vi "ReplaceScanFunc.vi"(0 "LoadedInstIn":refnum<class "BaseDevice.lvclass">[](array[class]), 1 "LoadedFuncArr":string[](array[string]), 2 "ScanFunc":string, 5 "ScanSubPan":refnum<vi>, 7 "WholeTask(No:T)":bool, 9 "ScanFuncArrIn":string[][](array[string]), 11 "ErrorIn(No Error)":errorcluster caption="entrée d'erreur (pas d'erreur)", 12 "ActScanPar":bool[](array[boolean]), 13 "TaskIdx":i32) -> (4 "LoadedInst":refnum<class "BaseDevice.lvclass">[](array[class]), 10 "ScanFuncArrOut":string[][](array[string]), 14 "ActScanParOut":bool[](array[boolean]), 15 "sortie d'erreur":errorcluster)   [LabVIEW 2019]
uses:
  DevicesClass/BaseDevice/BaseDevice.lvclass
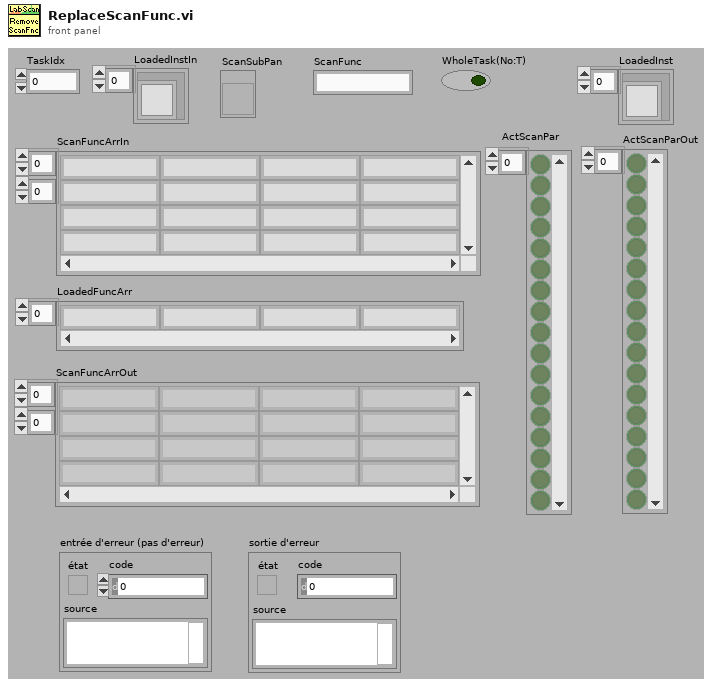
[diagram p1: front panel]
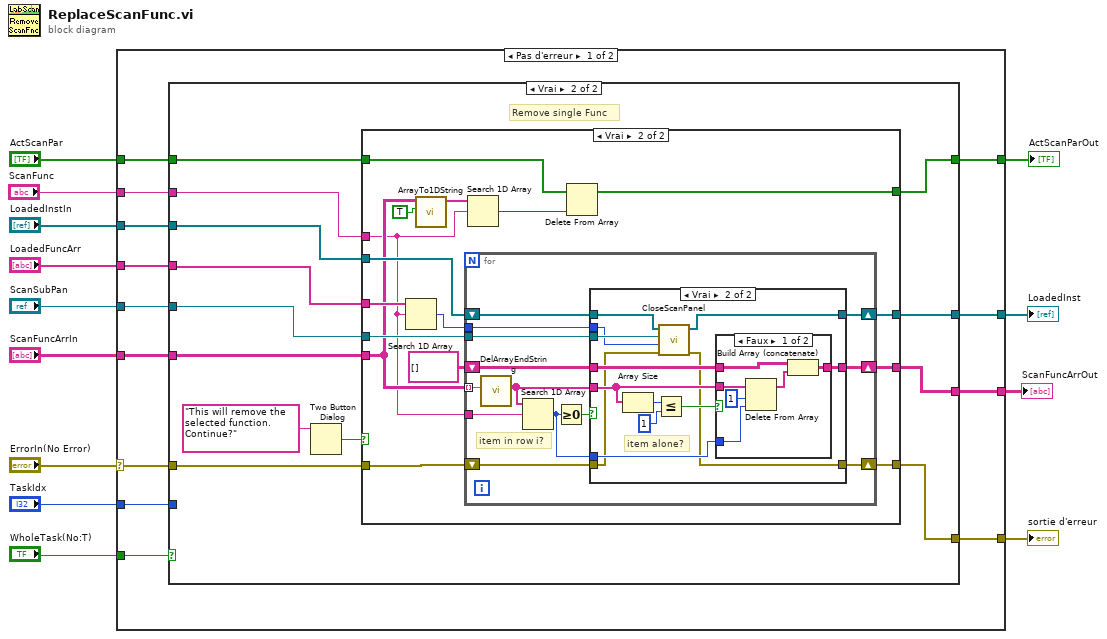
[diagram p0: block diagram]
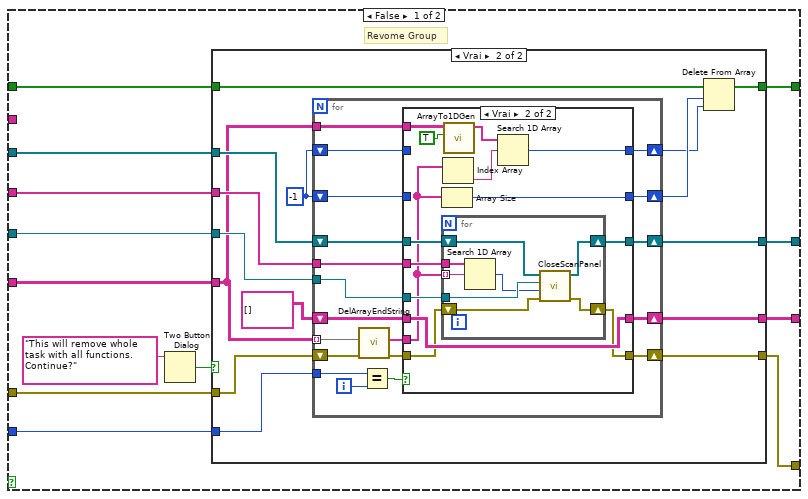
[diagram p2: hidden frame]
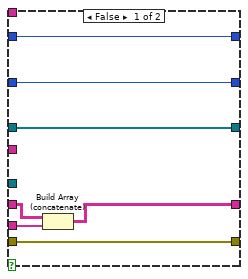
[diagram p4: hidden frame]
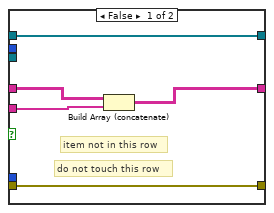
[diagram p6: hidden frame]
diagram:
  n1 = case shown="Pas d'erreur" "ErrorIn(No Error)" {
    selector: "ErrorIn(No Error)" -> [w26 w181]
    tunnel: "ScanFuncArrIn" -> [w23 w180]
    tunnel: "WholeTask(No:T)" -> [w24 _]
    tunnel: [w20 w181] -> w10
    tunnel: [w21 w180] -> w9
    tunnel: "ActScanPar" -> [w17 w179]
    tunnel: [w14 w179] -> w7
    tunnel: "TaskIdx" -> [w25 _]
    tunnel: [w22 w178] -> w5
    tunnel: "LoadedInstIn" -> [w19 w178]
    tunnel: "LoadedFuncArr" -> [w18 _]
    tunnel: "ScanSubPan" -> [w16 _]
    tunnel: "ScanFunc" -> [w15 _]
    frame No Error {
      n2 = case shown="Vrai" w24 {
        tunnel: w23 -> [w36 w116]
        tunnel: w25 -> [w35 _]
        tunnel: w17 -> [w28 w110]
        tunnel: w26 -> [w38 w112]
        tunnel: [w34 w119] -> w22
        tunnel: [w33 w118] -> w21
        tunnel: [w32 w117] -> w20
        tunnel: w19 -> [w30 w114]
        tunnel: w18 -> [w31 w113]
        tunnel: w16 -> [w29 w115]
        tunnel: w15 -> [_ w111]
        tunnel: [w27 w109] -> w14
        frame False {
          # "Revome Group"
          n3 = Two Button Dialog(message="This will remove whole task with all functions. Continue?") -> (T button?=w37:bool)  [unwired: 2 in]
          n4 = case shown="Vrai" w37 {
            tunnel: w36 -> [w43 w46]
            tunnel: w35 -> [_ w51]
            tunnel: [w43 w57] -> w33
            tunnel: w38 -> [w42 w58]
            tunnel: [w42 w56] -> w32
            tunnel: w30 -> [w41 w52]
            tunnel: w29 -> [_ w55]
            tunnel: w31 -> [_ w54]
            tunnel: [w41 w53] -> w34
            tunnel: w28 -> [w40 w50]
            tunnel: [w40 w48] -> w27
            frame False {
              # "canceled"
            }
            frame True {
              w45 = -1
              n5 = for {
                tunnel: w46 -> [w74] mode=indexing
                shift-right: [w70] -> w57
                shift-left: string[][] [] -> [w71]
                tunnel: w51 -> [w75]
                shift-right: [w69] -> w56
                shift-left: w58 -> [w77]
                tunnel: w55 -> [w67]
                tunnel: w54 -> [w66]
                shift-right: [w65] -> w53
                shift-left: w52 -> [w64]
                shift-right: [w63] -> w49
                shift-left: w45 -> [w62]
                tunnel: w46 -> [w61]
                shift-right: [w60] -> w44
                shift-left: w45 -> [w59]
                i -> [w76]
                n6 = call <userlib>:"DelArrayEndString.vi"("ErrorIn(No Error)"=w77, "Array In"=w74) -> ("sortie d'erreur"=w68:errorcluster, "Array Out"=w72:string[])  [unwired: 8 in]
                n7 = Equal?(x=w75, y=w76) -> (x = y?=w73:bool)
                n8 = case shown="Vrai" w73 {
                  tunnel: w72 -> [w84 w90]
                  tunnel: w71 -> [w83 w97]
                  tunnel: [w82 w97] -> w70
                  tunnel: [w81 w93] -> w69
                  tunnel: w68 -> [w81 w94]
                  tunnel: w64 -> [w80 w95]
                  tunnel: w67 -> [_ w96]
                  tunnel: w66 -> [_ w98]
                  tunnel: [w80 w92] -> w65
                  tunnel: [w79 w91] -> w63
                  tunnel: w62 -> [w79 _]
                  tunnel: w61 -> [_ w89]
                  tunnel: [w78 w85] -> w60
                  tunnel: w59 -> [w78 _]
                  frame False {
                    n9 = Build Array (concatenate)(w83, w84) -> (w82:string[][])
                  }
                  frame True {
                    n10 = Array Size(array=w90) -> (size(s)=w91:i32)
                    n11 = for {
                      tunnel: w98 -> [w99]
                      tunnel: w90 -> [w106] mode=indexing
                      tunnel: w96 -> [w103]
                      shift-right: [w104] -> w93
                      shift-left: w94 -> [w105]
                      shift-right: [w100] -> w92
                      shift-left: w95 -> [w101]
                      n12 = Search 1D Array(1D array=w99, element=w106) -> (index of element=w102:i32)  [unwired: 1 in]
                      n13 = call "CloseScanPanel.vi"("error in (no error)"=w105, "Index"=w102, "SubPanRef"=w103, "LoadedInst"=w101) -> ("sortie d'erreur"=w104:errorcluster, "LoadedInst Out"=w100:refnum<class "BaseDevice.lvclass">[])  [unwired: 6 in]
                    }
                    n14 = Index Array(array=w90) -> (element=w86:string)  [unwired: 1 in]
                    n15 = call-poly <userlib>:"ArrayTo1DGen.vi"("DelArrEnd(F)"=TRUE, "tableau"=w89) -> ("Array Out"=w87:string[])  [unwired: 7 in, 2 out]
                    n16 = Search 1D Array(1D array=w87, element=w86) -> (index of element=w85:i32)  [unwired: 1 in]
                  }
                }
              }
              n17 = Delete From Array(array=w50, length=w49, index=w44) -> (array with subset deleted=w48:bool[])  [unwired: 1 out]
            }
          }
        }
        frame True {
          # "Remove single Func"
          n18 = Two Button Dialog(message="This will remove the selected function. Continue?") -> (T button?=w107:bool)  [unwired: 2 in]
          n19 = case shown="Vrai" w107 {
            tunnel: w116 -> [w120 w131]
            tunnel: [w120 w138] -> w118
            tunnel: w111 -> [_ w129]
            tunnel: w114 -> [w123 w137]
            tunnel: w115 -> [_ w136]
            tunnel: w113 -> [_ w135]
            tunnel: [w121 w133] -> w117
            tunnel: [w123 w132] -> w119
            tunnel: w112 -> [w121 w128]
            tunnel: w110 -> [w122 w127]
            tunnel: [w122 w126] -> w109
            frame False {
              # "canceled"
            }
            frame True {
              n20 = Search 1D Array(1D array=w135, element=w129) -> (index of element=w134:i32)  [unwired: 1 in]
              n21 = call <userlib>:"ArrayTo1DString.vi"("DelArrEnd(F)"=TRUE, "tableau"=w131) -> ("Array Out"=w130:string[])  [unwired: 7 in, 2 out]
              n22 = for {
                tunnel: w131 -> [w150] mode=indexing
                tunnel: w129 -> [w152]
                shift-right: [w147] -> w138
                shift-left: string[][] [] -> [w148]
                tunnel: w136 -> [w145]
                tunnel: w134 -> [w143]
                shift-right: [w141] -> w133
                shift-left: w128 -> [w142]
                shift-right: [w140] -> w132
                shift-left: w137 -> [w146]
                # "item in row i?"
                n23 = call <userlib>:"DelArrayEndString.vi"("Array In"=w150) -> ("Array Out"=w149:string[])  [unwired: 9 in, 1 out]
                n24 = Search 1D Array(1D array=w149, element=w152) -> (index of element=w144:i32)  [unwired: 1 in]
                n25 = Greater Or Equal To 0?(x=w144) -> (x >= 0?=w151:bool)
                n26 = case shown="Vrai" w151 {
                  tunnel: [w156 w166] -> w147
                  tunnel: w149 -> [w157 w165]
                  tunnel: w148 -> [w155 w167]
                  tunnel: w146 -> [w153 w160]
                  tunnel: w145 -> [_ w163]
                  tunnel: w144 -> [_ w164]
                  tunnel: w143 -> [_ w159]
                  tunnel: w142 -> [w154 w162]
                  tunnel: [w154 w161] -> w141
                  tunnel: [w153 w158] -> w140
                  frame False {
                    # "item not in this row"
                    # "do not touch this row"
                    n27 = Build Array (concatenate)(w155, w157) -> (w156:string[][])
                  }
                  frame True {
                    # "item alone?"
                    n28 = Array Size(array=w165) -> (size(s)=w170:i32)
                    n29 = Less Or Equal?(x=w170, y=1) -> (x <= y?=w168:bool)
                    n30 = call "CloseScanPanel.vi"("error in (no error)"=w162, "Index"=w159, "SubPanRef"=w163, "LoadedInst"=w160) -> ("sortie d'erreur"=w161:errorcluster, "LoadedInst Out"=w158:refnum<class "BaseDevice.lvclass">[])  [unwired: 6 in]
                    n31 = case shown="Faux" w168 {
                      tunnel: w167 -> [w174 w177]
                      tunnel: [w172 w177] -> w166
                      tunnel: w165 -> [w175 _]
                      tunnel: w164 -> [w171 _]
                      frame False {
                        n32 = Delete From Array(array=w175, length=1 ("longueur"), index=w171) -> (array with subset deleted=w173:string[])  [unwired: 1 out]
                        n33 = Build Array (concatenate)(w174, w173) -> (w172:string[][])
                      }
                      frame True {
                        # "item not alone \ndelete row"
                      }
                    }
                  }
                }
              }
              n34 = Search 1D Array(1D array=w130, element=w129) -> (index of element=w125:i32)  [unwired: 1 in]
              n35 = Delete From Array(array=w127, index=w125) -> (array with subset deleted=w126:bool[])  [unwired: 1 in, 1 out]
            }
          }
        }
      }
    }
    frame Error {
    }
  }
  "sortie d'erreur" <- w10
  "ScanFuncArrOut" <- w9
  "ActScanParOut" <- w7
  "LoadedInst" <- w5
